vi "Diff_Drive_System_Acquire_Act.vi"(6 "FPGA_Time_Seconds":dbl, 11 "DiffDriveDeviceRefs":T1 {"GyroDevRef"."Sample Rate" min=0.25 max=100.0 step=0.25}) -> ()   [LabVIEW 2019]
uses:
  Diff_Drive_System_Device_Refs.ctl
  <vilib>/Rock Robotics/WPI/Gyro/WPI_GyroDevRef.ctl
  <vilib>/Rock Robotics/SystemInterfaces/AI/FPGA_AIChannel.ctl
  <vilib>/Rock Robotics/SystemInterfaces/spilib/spi_bus.ctl
  <vilib>/Rock Robotics/WPI/RobotDrive/WPI_RobotDriveDevRef.ctl
  <vilib>/Rock Robotics/WPI/MotorControl/WPI_MotorControlDeviceRef.ctl
  <vilib>/Rock Robotics/WPI/MotorControl/WPI_MotorControlType.ctl
  <vilib>/Rock Robotics/SystemInterfaces/DIO/FPGA_DIOPWMChannel.ctl
  <vilib>/Rock Robotics/WPI/PWM/WPI_PWMDeadband.ctl
  <vilib>/Rock Robotics/SystemInterfaces/DIO/FPGA_DIOChannel.ctl
  <vilib>/Rock Robotics/WPI/Encoder/WPI_EncoderDevRef.ctl
  <vilib>/Rock Robotics/SystemInterfaces/Encoder/FPGA_EncoderIdx.ctl
  <vilib>/Rock Robotics/SystemInterfaces/Counter/FPGA_CounterCtrSystemIndex.ctl
  <vilib>/Rock Robotics/WPI/Encoder/WPI_EncoderType.ctl
  <vilib>/Rock Robotics/WPI/ThirdParty/JAS_Junk/TrajLib/VI/BoolCmd_Recv_Internal.vi
  <vilib>/Rock Robotics/WPI/ThirdParty/JAS_Junk/TrajLib/VI/BoolCmd_ObtainQueue.vi
  Trajectory_Execution_Diff_Drive/Trajectory_Execution_Globals.vi
  Diff_Drive_System_Globals.vi
  <vilib>/Rock Robotics/WPI/ThirdParty/JAS_Junk/TrajLib/Trajectory_Library.lvlib
panel:
  # "Analog"
  # "XRS"
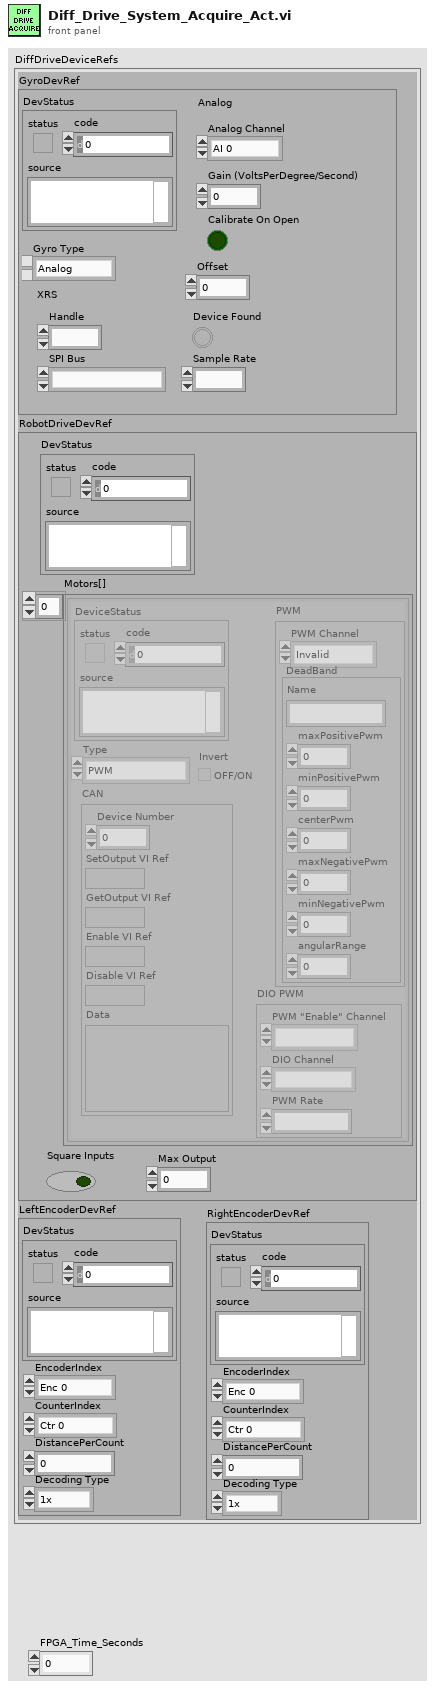
[diagram p1: front panel]
types:
  T1 = typedef "Diff_Drive_System_Device_Refs.ctl" = cluster{"GyroDevRef":T2, "RobotDriveDevRef":T5, "LeftEncoderDevRef":T11, "RightEncoderDevRef":T11}
  T2 = typedef "WPI_GyroDevRef.ctl" = cluster{"DevStatus":errorcluster, "Analog Channel":T3, "Gain (VoltsPerDegree/Second)":dbl, "Gyro Type":enum16{"Analog", "XRS450"}, "Handle":i32, "SPI Bus":T4, "Device Found":bool, "Sample Rate":dbl, "Calibrate On Open":bool, "Offset":dbl}
  T3 = typedef "FPGA_AIChannel.ctl" = enum8{"AI 0", "AI 1", "AI 2", "AI 3", "AI MXP 0", "AI MXP 1", "AI MXP 2", "AI MXP 3", "Invalid"}
  T4 = typedef "spi_bus.ctl" = enum16{"SPI On-Board, CS0", "SPI On-Board, CS1", "SPI On-Board, CS2", "SPI On-Board, CS3", "SPI MXP", "Invalid"}
  T5 = typedef "WPI_RobotDriveDevRef.ctl" = cluster{"DevStatus":errorcluster, "Motors[]":T6[], "Square Inputs":bool, "Max Output":dbl}
  T6 = typedef "WPI_MotorControlDeviceRef.ctl" = cluster{"DeviceStatus":errorcluster, "Type":T7, "PWM":cluster{"PWM Channel":T8, "DeadBand":T9}, "CAN":cluster{"Device Number":u8, "SetOutput VI Ref":variant, "GetOutput VI Ref":variant, "Enable VI Ref":variant, "Disable VI Ref":variant, "Data":variant}, "Invert":bool, "DIO PWM":cluster{"PWM \"Enable\" Channel":T8, "DIOChannel":T10, "PWM Rate":dbl}}
  T7 = typedef "WPI_MotorControlType.ctl" = enum16{"PWM", "CAN", "DIO PWM"}
  T8 = typedef "FPGA_DIOPWMChannel.ctl" = enum8{"PWM 0", "PWM 1", "PWM 2", "PWM 3", "PWM 4", "PWM 5", "PWM 6", "PWM 7", "PWM 8", "PWM 9", "PWM MXP 0", "PWM MXP 1", "PWM MXP 2", "PWM MXP 3", "PWM MXP 4", "PWM MXP 5", "PWM MXP 6", "PWM MXP 7", "PWM MXP 8", "PWM MXP 9", "Invalid"}
  T9 = typedef "WPI_PWMDeadband.ctl" = cluster{"Name":string, "maxPositivePwm":i32, "minPositivePwm":i32, "centerPwm":i32, "maxNegativePwm":i32, "minNegativePwm":i32, "angularRange":u16}
  T10 = typedef "FPGA_DIOChannel.ctl" = enum8{"DIO 0", "DIO 1", "DIO 2", "DIO 3", "DIO 4", "DIO 5", "DIO 6", "DIO 7", "DIO 8", "DIO 9", "DIO MXP 0", "DIO MXP 1", "DIO MXP 2", "DIO MXP 3", "DIO MXP 4", "DIO MXP 5", "DIO MXP 6", "DIO MXP 7", "DIO MXP 8", "DIO MXP 9", "DIO MXP 10", "DIO MXP 11", "DIO MXP 12", "DIO MXP 13", "DIO MXP 14", "DIO MXP 15", "SPI Port CS1", "SPI Port CS2", "SPI Port CS3", "SPI Port MISO", "SPI Port MOSI", "Invalid"}
  T11 = typedef "WPI_EncoderDevRef.ctl" = cluster{"DevStatus":errorcluster, "EncoderIndex":T12, "CounterIndex":T13, "DistancePerCount":dbl, "Decoding Type":T14}
  T12 = typedef "FPGA_EncoderIdx.ctl" = enum8{"Enc 0", "Enc 1", "Enc 2", "Enc 3", "Enc 4", "Enc 5", "Enc 6", "Enc 7", "Invalid"}
  T13 = typedef "FPGA_CounterCtrSystemIndex.ctl" = enum8{"Ctr 0", "Ctr 1", "Ctr 2", "Ctr 3", "Ctr 4", "Ctr 5", "Ctr 6", "Ctr 7", "Invalid"}
  T14 = typedef "WPI_EncoderType.ctl" = enum16{"1x", "2x", "4x"}
  T15 = typedef "Trajectory_Library.lvlib/SIMPLE_MOTOR_FF.ctl" = cluster{"Ks":dbl, "Kv":dbl, "Ka":dbl, "KnInv":dbl}
  T16 = typedef "Trajectory_Library.lvlib/PID_ADV_LIMITS.ctl" = cluster{"MaxInput":dbl, "MinInput":dbl, "Continuous":bool, "MaxOutput":dbl, "MinOutput":dbl}
  T17 = typedef "Trajectory_Library.lvlib/PID_ADV_TUNING.ctl" = cluster{"Kf":dbl, "Kp":dbl, "Ki":dbl, "Kd":dbl, "MaximumIntegral":dbl, "MinimumIntegral":dbl, "Filter Derivative":bool}
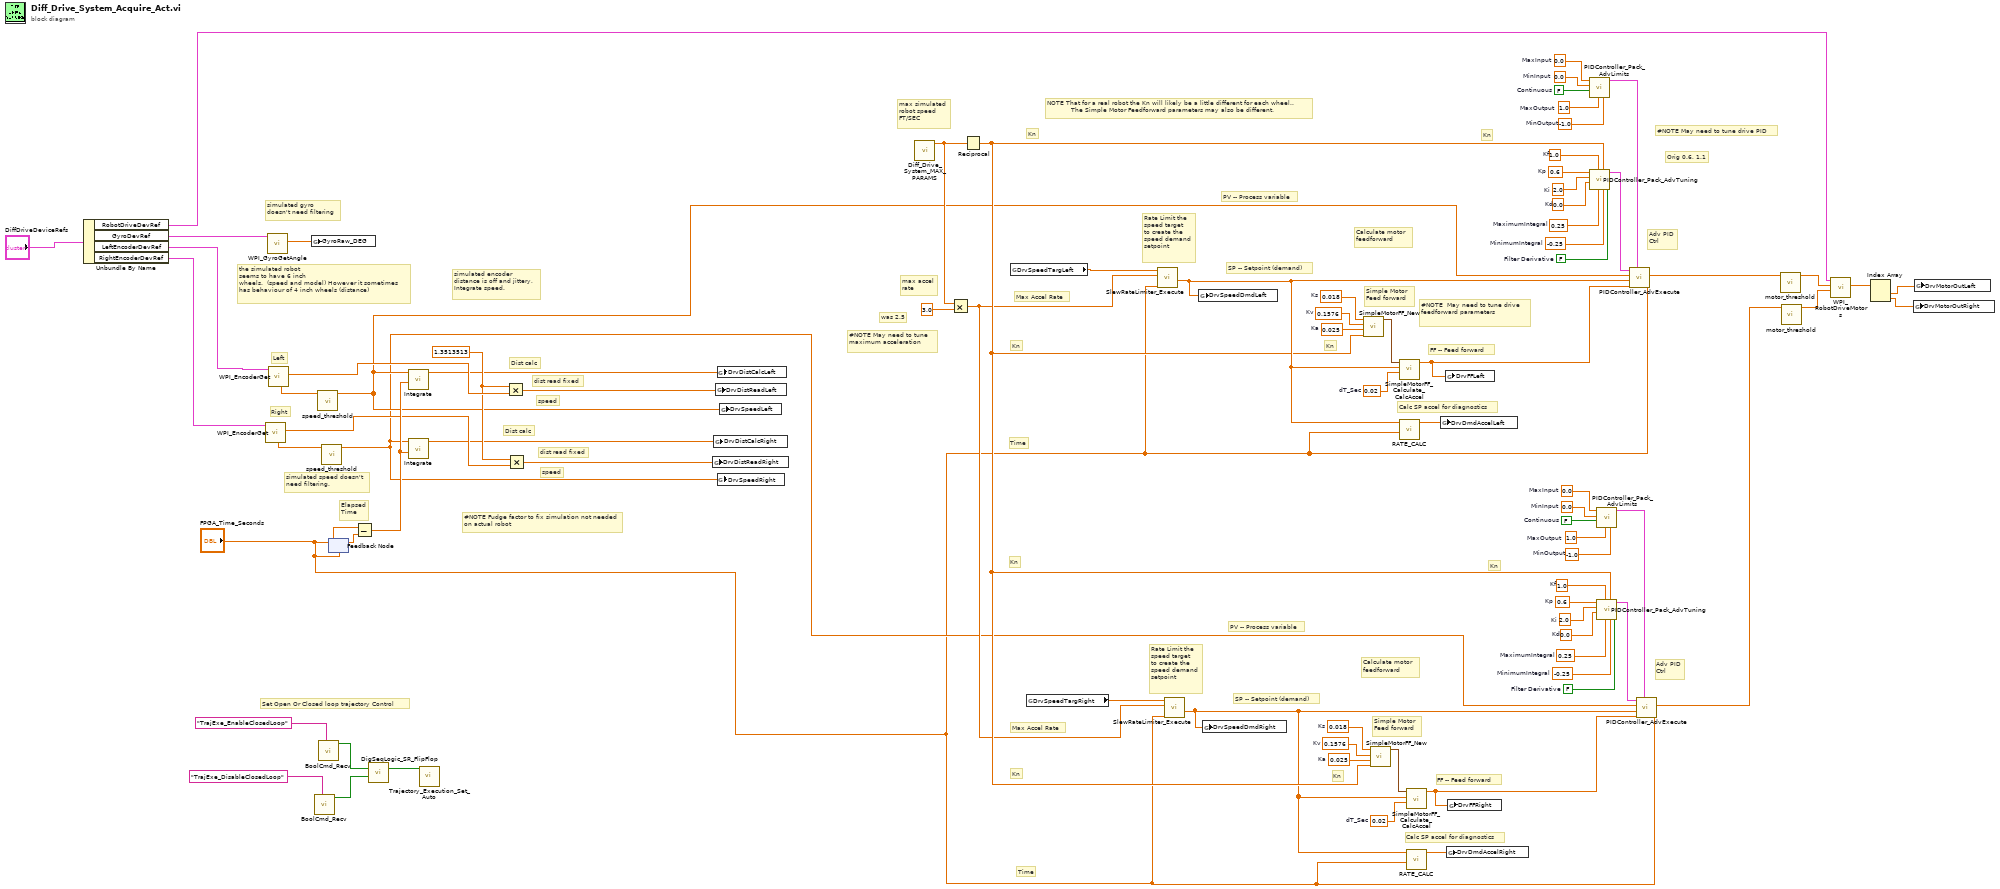
[diagram p0: block diagram]
diagram:
  w25 = 0.6  # Kp
  w24 = 2.0  # Ki
  w23 = 0.0  # Kd
  w22 = 1.0  # Kf
  w21 = 0.25  # MaximumIntegral
  w20 = -0.25  # MinimumIntegral
  w19 = FALSE  # Filter Derivative
  w17 = 0.0  # MinInput
  w16 = FALSE  # Continuous
  w15 = 1.0  # MaxOutput
  w18 = -1.0  # MinOutput
  w14 = 0.0  # MaxInput
  w30 = 0.02  # dT_Sec
  w28 = 0.018  # Ks
  w27 = 0.1576  # Kv
  w26 = 0.025  # Ka
  w49 = 0.6  # Kp
  w48 = 2.0  # Ki
  w47 = 0.0  # Kd
  w46 = 1.0  # Kf
  w45 = 0.25  # MaximumIntegral
  w44 = -0.25  # MinimumIntegral
  w43 = FALSE  # Filter Derivative
  w41 = 0.0  # MinInput
  w40 = FALSE  # Continuous
  w39 = 1.0  # MaxOutput
  w42 = -1.0  # MinOutput
  w38 = 0.0  # MaxInput
  w55 = 0.02  # dT_Sec
  w53 = 0.018  # Ks
  w52 = 0.1576  # Kv
  w51 = 0.025  # Ka
  w76 = 1.3513513
  # "Orig 0.6, 1.1"
  # "NOTE That for a real robot the Kn will likely be a little different for each wheel..\n            The Simple Motor Feedforward parameters may also be different."
  # "Max Accel Rate"
  # "Max Accel Rate"
  # "Time"
  # "Kn"
  # "Kn"
  # "Kn"
  # "Kn"
  # "Time"
  # "Kn"
  # "PV -- Process variable"
  # "Kn"
  # "Calc SP accel for diagnostics"
  # "FF -- Feed forward"
  # "SP -- Setpoint (demand)"
  # "Adv PID\nCtrl"
  # "Calculate motor\nfeedforward"
  # "Rate Limit the \nspeed target\nto create the\nspeed demand\nsetpoint"
  # "Simple Motor\nFeed forward"
  # "Kn"
  # "PV -- Process variable"
  # "Kn"
  # "Calc SP accel for diagnostics"
  # "FF -- Feed forward"
  # "SP -- Setpoint (demand)"
  # "Adv PID\nCtrl"
  # "Calculate motor\nfeedforward"
  # "was 2.5"
  # "Rate Limit the \nspeed target\nto create the\nspeed demand\nsetpoint"
  # "Simple Motor\nFeed forward"
  # "#NOTE May need to tune drive PID"
  # "#NOTE May need to tune maximum acceleration"
  # "#NOTE  May need to tune drive feedforward parameters"
  # "max simulated\nrobot speed\nFT/SEC"
  # "max accel\nrate"
  # "Set Open Or Closed loop trajectory Control"
  # "#NOTE Fudge factor to fix simulation not needed on actual robot"
  # "Elapsed\nTime"
  # "simulated speed doesn't\nneed filtering."
  # "simulated gyro \ndoesn't need filtering"
  # "Right"
  # "Left"
  # "the simulated robot\nseems to have 6 inch\nwheels.  (speed and model) However it sometimes\nhas behaviour of 4 inch wheels (distance)"
  # "speed"
  # "dist read fixed"
  # "Dist calc"
  # "speed"
  # "dist read fixed"
  # "Dist calc"
  # "simulated encoder\ndistance is off and jittery,\nIntegrate speed."
  n1 = Unbundle By Name("DiffDriveDeviceRefs") -> ("RobotDriveDevRef"=w4:T5, "GyroDevRef"=w69:T2, "LeftEncoderDevRef"=w68:T11, "RightEncoderDevRef"=w67:T11)
  n2 = call <vilib>:"WPI_EncoderGet.vi"("EncoderDevRef"=w67) -> ("Distance"=w78:dbl, "Rate"=w80:dbl)  [unwired: 5 in, 4 out]
  n3 = call <vilib>:"WPI_GyroGetAngle.vi"("GyroDevRef"=w69) -> ("Angle"=w75:dbl)  [unwired: 6 in, 4 out]
  n4 = call <vilib>:"WPI_EncoderGet.vi"("EncoderDevRef"=w68) -> ("Distance"=w77:dbl, "Rate"=w79:dbl)  [unwired: 5 in, 4 out]
  n5 = global write "Diff_Drive_System_Globals.vi" "GyroRaw_DEG"(w75) -> ()
  n6 = call <vilib>:"BoolCmd_Recv.vi"("Command Name"="TrajExe_DisableClosedLoop") -> ("New Request"=w63:bool)  [unwired: 9 in, 1 out]
  n7 = call "speed_threshold.vi"("SPEED IN"=w79) -> ("SPEED OUT"=w3:dbl)  [unwired: 10 in]
  n8 = call <vilib>:"BoolCmd_Recv.vi"("Command Name"="TrajExe_EnableClosedLoop") -> ("New Request"=w64:bool)  [unwired: 9 in, 1 out]
  n9 = call "speed_threshold.vi"("SPEED IN"=w80) -> ("SPEED OUT"=w2:dbl)  [unwired: 10 in]
  n10 = feedback #1("FPGA_Time_Seconds") -> (w81:dbl)
  n11 = feedback-in #1("FPGA_Time_Seconds") -> ()
  n12 = Subtract(x="FPGA_Time_Seconds", y=w81) -> (x-y=w82:dbl)
  n13 = call <vilib>:"DigSeqLogic_SR_FlipFlop.vi"("Set"=w64, "Reset"=w63) -> ("Output"=w62:bool)  [unwired: 12 in, 1 out]
  n14 = call "Integrate.vi"("Elapsed Sec"=w82, "Rate"=w3) -> ("DIST"=w74:dbl)  [unwired: 9 in]
  n15 = call "Integrate.vi"("Elapsed Sec"=w82, "Rate"=w2) -> ("DIST"=w72:dbl)  [unwired: 9 in]
  n16 = call "Trajectory_Execution_Set_Auto.vi"("Ramsete AUTO"=w62) -> ()  [unwired: 11 in]
  n17 = Multiply(x=w76, y=w77) -> (x*y=w73:dbl)
  n18 = Multiply(x=w76, y=w78) -> (x*y=w71:dbl)
  n19 = global write "Diff_Drive_System_Globals.vi" "DrvDistReadRight"(w71) -> ()
  n20 = global write "Diff_Drive_System_Globals.vi" "DrvDistCalcRight"(w72) -> ()
  n21 = global write "Diff_Drive_System_Globals.vi" "DrvDistReadLeft"(w73) -> ()
  n22 = global write "Diff_Drive_System_Globals.vi" "DrvDistCalcLeft"(w74) -> ()
  n23 = global write "Diff_Drive_System_Globals.vi" "DrvSpeedRight"(w2) -> ()
  n24 = global write "Diff_Drive_System_Globals.vi" "DrvSpeedLeft"(w3) -> ()
  n25 = call "Diff_Drive_System_MAX_PARAMS.vi"() -> ("Max Speed Ft/Sec"=w33:dbl)  [unwired: 10 in, 1 out]
  n26 = Multiply(x=w33, y=3.0 ("x")) -> (x*y=w9:dbl)
  n27 = Reciprocal(x=w33) -> (1/x=w10:dbl)
  n28 = global read "Diff_Drive_System_Globals.vi" "DrvSpeedTargLeft"() -> (w50:dbl)
  n29 = global read "Diff_Drive_System_Globals.vi" "DrvSpeedTargRight"() -> (w8:dbl)
  n30 = call <vilib>:"SlewRateLimiter_Execute.vi"("Time"="FPGA_Time_Seconds", "PositiveRate"=w9, "Input"=w50) -> ("Output"=w35:dbl)  [unwired: 7 in, 1 out]
  n31 = call <vilib>:"SlewRateLimiter_Execute.vi"("Time"="FPGA_Time_Seconds", "PositiveRate"=w9, "Input"=w8) -> ("Output"=w5:dbl)  [unwired: 7 in, 1 out]
  n32 = global write "Diff_Drive_System_Globals.vi" "DrvSpeedDmdLeft"(w35) -> ()
  n33 = global write "Diff_Drive_System_Globals.vi" "DrvSpeedDmdRight"(w5) -> ()
  n34 = call <vilib>:"SimpleMotorFF_New.vi"("Kn"=w10, "Ka"=w51, "Kv"=w52, "Ks"=w53) -> ("SIMPLE_MOTOR_FF"=w54:T15)  [unwired: 7 in]
  n35 = call <vilib>:"SimpleMotorFF_New.vi"("Kn"=w10, "Ka"=w26, "Kv"=w27, "Ks"=w28) -> ("SIMPLE_MOTOR_FF"=w29:T15)  [unwired: 7 in]
  n36 = call <vilib>:"SimpleMotorFF_Calculate_CalcAccel.vi"("dT_Sec"=w55, "VelSp"=w35, "SIMPLE_MOTOR_FF"=w54) -> ("FeedForward"=w32:dbl)  [unwired: 8 in]
  n37 = call "RATE_CALC.vi"("Time"="FPGA_Time_Seconds", "Input"=w35) -> ("Output"=w34:dbl)  [unwired: 9 in]
  n38 = call <vilib>:"SimpleMotorFF_Calculate_CalcAccel.vi"("dT_Sec"=w30, "VelSp"=w5, "SIMPLE_MOTOR_FF"=w29) -> ("FeedForward"=w7:dbl)  [unwired: 8 in]
  n39 = call "RATE_CALC.vi"("Time"="FPGA_Time_Seconds", "Input"=w5) -> ("Output"=w6:dbl)  [unwired: 9 in]
  n40 = global write "Diff_Drive_System_Globals.vi" "DrvDmdAccelLeft"(w34) -> ()
  n41 = global write "Diff_Drive_System_Globals.vi" "DrvFFLeft"(w32) -> ()
  n42 = global write "Diff_Drive_System_Globals.vi" "DrvDmdAccelRight"(w6) -> ()
  n43 = global write "Diff_Drive_System_Globals.vi" "DrvFFRight"(w7) -> ()
  n44 = call <vilib>:"PIDController_Pack_AdvLimits.vi"("MinOutput"=w42, "MaxOutput"=w39, "Continuous"=w40, "MinInput"=w41, "MaxInput"=w38) -> ("Adv PID Limits"=w36:T16)  [unwired: 6 in]
  n45 = call <vilib>:"PIDController_Pack_AdvTuning.vi"("Filter Derivative"=w43, "MinimumIntegral"=w44, "Kn"=w10, "MaximumIntegral"=w45, "Kf"=w46, "Kd"=w47, "Ki"=w48, "Kp"=w49) -> ("Adv PID Tuning"=w37:T17)  [unwired: 3 in]
  n46 = call <vilib>:"PIDController_Pack_AdvLimits.vi"("MinOutput"=w18, "MaxOutput"=w15, "Continuous"=w16, "MinInput"=w17, "MaxInput"=w14) -> ("Adv PID Limits"=w12:T16)  [unwired: 6 in]
  n47 = call <vilib>:"PIDController_Pack_AdvTuning.vi"("Filter Derivative"=w19, "MinimumIntegral"=w20, "Kn"=w10, "MaximumIntegral"=w21, "Kf"=w22, "Kd"=w23, "Ki"=w24, "Kp"=w25) -> ("Adv PID Tuning"=w13:T17)  [unwired: 3 in]
  n48 = call <vilib>:"PIDController_AdvExecute.vi"("Time"="FPGA_Time_Seconds", "Adv PID Limits"=w36, "FF-FeedForward"=w32, "SP-SetPoint"=w35, "PV-Measurement"=w3, "Adv PID Tuning"=w37) -> ("CO-ControlOutput"=w31:dbl)  [unwired: 3 in, 2 out]
  n49 = call <vilib>:"PIDController_AdvExecute.vi"("Time"="FPGA_Time_Seconds", "Adv PID Limits"=w12, "FF-FeedForward"=w7, "SP-SetPoint"=w5, "PV-Measurement"=w2, "Adv PID Tuning"=w13) -> ("CO-ControlOutput"=w11:dbl)  [unwired: 3 in, 2 out]
  n50 = call "motor_threshold.vi"("motor in"=w31) -> ("motor out"=w59:dbl)  [unwired: 10 in]
  n51 = call "motor_threshold.vi"("motor in"=w11) -> ("motor out"=w60:dbl)  [unwired: 10 in]
  n52 = call <vilib>:"WPI_RobotDriveMotors.vi"("RightSpeed"=w60, "LeftSpeed"=w59, "RobotDriveDevRef"=w4) -> ("Motor Values"=w58:dbl[])  [unwired: 6 in, 2 out]
  n53 = Index Array(array=w58) -> (element #1=w57:dbl, element #2=w56:dbl)  [unwired: 2 in]
  n54 = global write "Diff_Drive_System_Globals.vi" "DrvMotorOutRight"(w56) -> ()
  n55 = global write "Diff_Drive_System_Globals.vi" "DrvMotorOutLeft"(w57) -> ()
